vi "Begin V.3.0.vi"(8 "error in":errorcluster) -> (0 "error out":errorcluster)   [LabVIEW 2017]
doc: "Called before other user functions, this VI is expected to open initial I/O refnums, load in file data, and do all program initialization. Notice that the <B>error out</B> terminal is simply used for data flow. Wiring it to other structures or subVIs ensures that this VI runs first."
uses:
  <vilib>/Rock Robotics/WPI/DriverStation/WPI_DriverStationRobotMode2.ctl
  Robot Global Data V.3.0.vi
  <vilib>/Rock Robotics/Network Tables/NT Write String Array.vi
  <vilib>/Rock Robotics/Network Tables/NT Write Boolean.vi
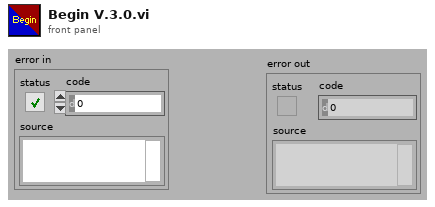
[diagram p1: front panel]
types:
  T1 = cluster{"Pot. Voltage":dbl[], "Corresponding Inches":dbl[]}
  T2 = typedef "WPI_DriverStationRobotMode2.ctl" = enum16{"Autonomous Disabled", "Autonomous Enabled", "Teleop Disabled", "Teleop Enabled", "Disconnected", "Finish", "Test Disabled", "Test Enabled", "Emergency Stopped"}
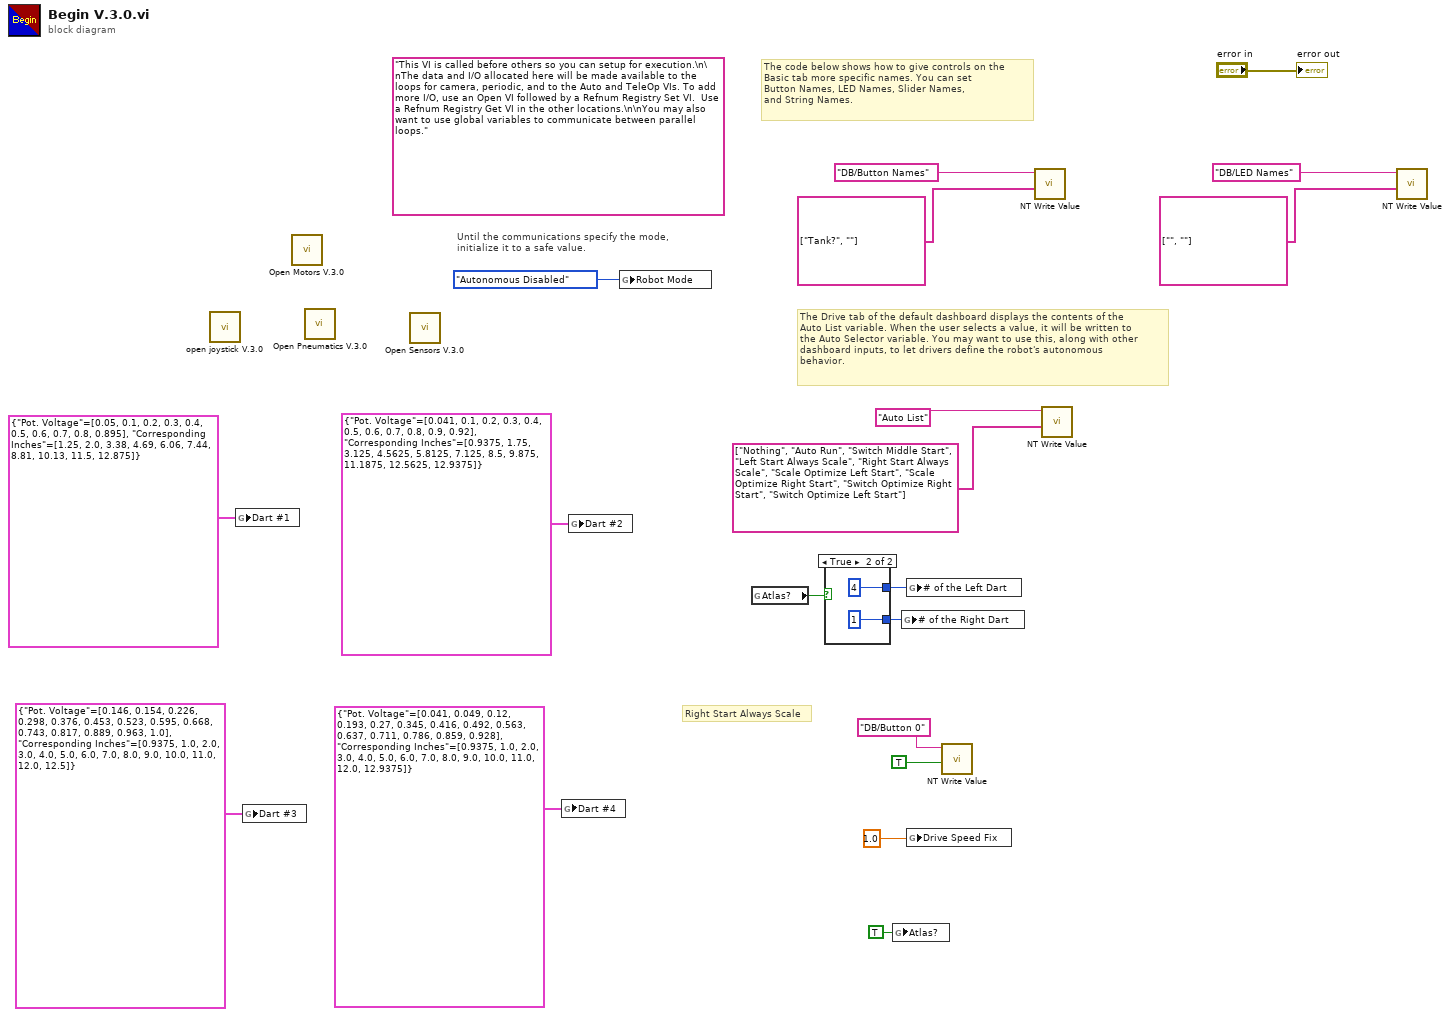
[diagram p0: block diagram]
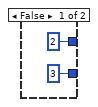
[diagram p2: hidden frame]
diagram:
  (unwired) "This VI is called before others so you can setup for execution.\n\nThe data and I/O allocated here will be made available to the loops for camera, periodic, and to the Auto and TeleOp VIs. To add more I/O, use an Open VI followed by a Refnum Registry Set VI.  Use a Refnum Registry Get VI in the other locations.\n\nYou may also want to use global variables to communicate between parallel loops."
  # "Right Start Always Scale"
  # "The Drive tab of the default dashboard displays the contents of the\nAuto List variable. When the user selects a value, it will be written to\nthe Auto Selector variable. You may want to use this, along with other\ndashboard inputs, to let drivers define the robot's autonomous\nbehavior."
  # "The code below shows how to give controls on the\nBasic tab more specific names. You can set\nButton Names, LED Names, Slider Names,\nand String Names."
  # "Until the communications specify the mode,\ninitialize it to a safe value."
  n1 = call "open joystick V.3.0.vi"() -> ()  [unwired: 12 in]
  n2 = global write "Robot Global Data V.3.0.vi" "Dart #1"(T1 {"Pot. Voltage"=[0.05, 0.1, 0.2, 0.3, 0.4, 0.5, 0.6, 0.7, 0.8, 0.895], "Corresponding Inches"=[1.25, 2.0, 3.38, 4.69, 6.06, 7.44, 8.81, 10.13, 11.5, 12.875]}) -> ()
  n3 = global write "Robot Global Data V.3.0.vi" "Dart #3"(T1 {"Pot. Voltage"=[0.146, 0.154, 0.226, 0.298, 0.376, 0.453, 0.523, 0.595, 0.668, 0.743, 0.817, 0.889, 0.963, 1.0], "Corresponding Inches"=[0.9375, 1.0, 2.0, 3.0, 4.0, 5.0, 6.0, 7.0, 8.0, 9.0, 10.0, 11.0, 12.0, 12.5]}) -> ()
  n4 = call "Open Motors V.3.0.vi"() -> ()  [unwired: 12 in]
  n5 = call "Open Pneumatics V.3.0.vi"() -> ()  [unwired: 12 in]
  n6 = call "Open Sensors V.3.0.vi"() -> ()  [unwired: 12 in]
  n7 = global write "Robot Global Data V.3.0.vi" "Dart #4"(T1 {"Pot. Voltage"=[0.041, 0.049, 0.12, 0.193, 0.27, 0.345, 0.416, 0.492, 0.563, 0.637, 0.711, 0.786, 0.859, 0.928], "Corresponding Inches"=[0.9375, 1.0, 2.0, 3.0, 4.0, 5.0, 6.0, 7.0, 8.0, 9.0, 10.0, 11.0, 12.0, 12.9375]}) -> ()
  n8 = global write "Robot Global Data V.3.0.vi" "Dart #2"(T1 {"Pot. Voltage"=[0.041, 0.1, 0.2, 0.3, 0.4, 0.5, 0.6, 0.7, 0.8, 0.9, 0.92], "Corresponding Inches"=[0.9375, 1.75, 3.125, 4.5625, 5.8125, 7.125, 8.5, 9.875, 11.1875, 12.5625, 12.9375]}) -> ()
  n9 = global write "Robot Global Data V.3.0.vi" "Robot Mode"(WPI_DriverStationRobotMode2."Autonomous Disabled" ("Robot Mode")) -> ()
  n10 = global read "Robot Global Data V.3.0.vi" "Atlas?"() -> (w1:bool)
  n11 = case shown="True" w1 {
    tunnel: [2 4] -> w4
    tunnel: [3 1] -> w3
    frame False {
    }
    frame True {
    }
  }
  n12 = global write "Robot Global Data V.3.0.vi" "Atlas?"(TRUE ("Atlas?")) -> ()
  n13 = global write "Robot Global Data V.3.0.vi" "# of the Right Dart"(w3) -> ()
  n14 = global write "Robot Global Data V.3.0.vi" "# of the Left Dart"(w4) -> ()
  n15 = global write "Robot Global Data V.3.0.vi" "Drive Speed Fix"(1.0) -> ()
  n16 = call-poly <vilib>:"NT Write Value.vi"("Boolean"=TRUE, "Name"="DB/Button 0") -> ()  [unwired: 9 in, 1 out]
  n17 = call-poly <vilib>:"NT Write Value.vi"("String Array"=string[] ["Tank?", ""], "Name"="DB/Button Names") -> ()  [unwired: 9 in, 1 out]
  n18 = call-poly <vilib>:"NT Write Value.vi"("String Array"=string[] ["Nothing", "Auto Run", "Switch Middle Start", "Left Start Always Scale", "Right Start Always Scale", "Scale Optimize Left Start", "Scale Optimize Right Start", "Switch Optimize Right Start", "Switch Optimize Left Start"], "Name"="Auto List") -> ()  [unwired: 9 in, 1 out]
  n19 = call-poly <vilib>:"NT Write Value.vi"("String Array"=string[] ["", ""], "Name"="DB/LED Names") -> ()  [unwired: 9 in, 1 out]
  "error out" <- "error in"
